vi "Settings_Config.vi"(11 "DataCluster in":T1={"Core"={"Current VI Reference"=refnum, "Close Panel on Exit?"=FALSE, "Exit"=FALSE, "Initialized?"=TRUE}, "Connections"={"cDAQ"={"Task"="", "Connected"=FALSE, "Active"=FALSE, "ID"="N/A"}, "Camera"={"Session"="", "Connected"=FALSE, "Active"=FALSE, "Placeholder"="remote image 00000211C32F1B68"}, "PSU"={"Port"="", "Connected"=FALSE, "Active"=FALSE}, "Arduino"={"Port"="", "Connected"=FALSE, "Active"=FALSE}}, "Data Acquisition"={"Setup"={"Label"="Sample_5", "Operator"="N/A", "Notes"="", "TempGrad"=-1.0, "TargetTemp"=-30.0, "Sample Volume"=1.0}, "Camera"={"Image"=refnum, "Save Image"=refnum, "Image Frequency"=20, "Rectangle"={"Left"=0, "Top"=0, "Right"=480, "Bottom"=620, "Rotation"=0.0}, "Calibration"={"Top Left"={"X"=62.0, "Y"=65.0}, "Top Right"={"X"=420.0, "Y"=58.0}, "Bottom Left"={"X"=67.0, "Y"=299.0}, "Bottom Right"={"X"=425.0, "Y"=292.0}, "Fixpoint"={"X"=469.0, "Y"=23.0}, "Scan Area"=5.0, "Fixpoint Area"=5.0, "Well Pixels"=array384x29[11136 elements], "Valid"=TRUE}, "FocusPos"=33419, "Display Mapping"=15, "Camera Mode"=10}, "Thermistor"={"Sample Size"=30, "Calibration"={"B0.100"=[3749.4, 3749.4, 3746.6, 3750.1, 3743.8, 3741.2, 3742.3, 3742.5], "R25"=[2.2631, 2.2631, 2.2535, 2.2652, 2.2631, 2.2501, 2.2549, 2.2676], "c"=[[-2.06472, 1.37415, -0.319461, 0.0344214, -0.0014593], [-2.06472, 1.37415, -0.319461, 0.0344214, -0.0014593], [-1.73592, 1.09563, -0.233459, 0.0229947, -0.0009224], [-2.12763, 1.40062, -0.319406, 0.0337046, -0.0014085], [-2.17313, 1.44996, -0.337063, 0.036201, -0.0015282], [-2.0427871, 1.4165762, -0.345474, 0.0385267, -0.0016538], [-2.1725266, 1.4989325, -0.3661616, 0.0412033, -0.0017892], [-2.2048521, 1.4601067, -0.3370514, 0.0360935, -0.0015259]], "State"=[FALSE, TRUE, TRUE, FALSE, TRUE, FALSE, FALSE, FALSE], "V_S"=12.004, "R_S"=10.0}, "Timing Mode"=14712}, "Partition"={"Data"=[["A", "35%", "", "", ""], ["B", "15%", "", "", ""], ["C", "5%", "", "", ""], ["D", "35%", "", "", ""], ["E", "Test sample", "", "", ""], ["F", "High Concentration", "", "", ""], ["G", "Low Concentration", "", "", ""], ["X", "Empty", "", "", ""]], "Cell Label"="A", "Cell Color"=29373, "Height"=10, "Width"=16, "Grid"=[]}, "Queue"={"Size"=10, "Queue"=refnum}, "Sample Rate"=120, "Active"=FALSE, "Ready"=TRUE, "Graph Mode"=0, "Gradient Buffer"=10}, "Control"={"Sample Rate"=1, "PID gains"={"proportional gain (Kc)"=6.485, "integral time (Ti, min)"=0.09, "derivative time (Td, min)"=0.03}}, "Manual Temp Control"={"TargetTemp"=1.0, "Mode"=0, "Active"=FALSE}} {"Manual Temp Control"."Mode" items=["Cool", "Heat"]; "Manual Temp Control"."TargetTemp" min=-40.0 max=40.0 step=0.5 format="%#_g °C"; "Control"."PID gains"."derivative time (Td, min)" format="%.3f"; "Control"."PID gains"."integral time (Ti, min)" format="%.3f"; "Control"."PID gains"."proportional gain (Kc)" format="%.3f"; "Control"."Sample Rate" min=1 max=20 step=1 format="%.0f Samples/sec"; "Data Acquisition"."Gradient Buffer" min=2 max=30 step=1; "Data Acquisition"."Graph Mode" items=["Thermistor Temperature", "Camera Temperature"]; "Data Acquisition"."Thermistor"."Timing Mode" items=["Automatic"=16097, "High Resolution"=10195, "High Speed"=14712, "Best 50 Hz Rejection"=14713, "Best 60 Hz Rejection"=14714, "Custom"=10137]; "Data Acquisition"."Thermistor"."Calibration"."R_S" min=0.1 max=1000.0 format="%#_g kOhm"; "Data Acquisition"."Thermistor"."Calibration"."V_S" min=5.0 max=48.0 format="%#_g V"; "Data Acquisition"."Thermistor"."Calibration"."R25" min=0.1 max=1000.0 format="%#_g kOhm"; "Data Acquisition"."Thermistor"."Calibration"."B0.100" min=100.0 max=10000.0 format="%#_g K"; "Data Acquisition"."Thermistor"."Sample Size" min=1 max=200; "Data Acquisition"."Sample Rate" min=20 max=240 format="%.0f samples/min"; "Data Acquisition"."Queue"."Size" min=1 max=200; "Data Acquisition"."Camera"."Camera Mode" items=["Temperature Linear", "Signal Linear"]; "Data Acquisition"."Camera"."Display Mapping" items=["Default"=10, "Most Significant Bits"=11, "Full Dynamic"=12, "Downshift"=13, "Given Range"=14, "90% Dynamic"=15, "Given Percent Range"=16]; "Data Acquisition"."Camera"."Calibration"."Fixpoint"."Y" format="%.2f"; "Data Acquisition"."Camera"."Calibration"."Fixpoint"."X" format="%.2f"; "Data Acquisition"."Camera"."Calibration"."Top Left"."Y" format="%.2f"; "Data Acquisition"."Camera"."Calibration"."Top Left"."X" format="%.2f"; "Data Acquisition"."Camera"."Calibration"."Top Right"."Y" format="%.2f"; "Data Acquisition"."Camera"."Calibration"."Top Right"."X" format="%.2f"; "Data Acquisition"."Camera"."Calibration"."Bottom Left"."Y" format="%.2f"; "Data Acquisition"."Camera"."Calibration"."Bottom Left"."X" format="%.2f"; "Data Acquisition"."Camera"."Calibration"."Bottom Right"."Y" format="%.2f"; "Data Acquisition"."Camera"."Calibration"."Bottom Right"."X" format="%.2f"; "Data Acquisition"."Camera"."Rectangle"."Rotation" min=-90.0 max=90.0 step=1.0 format="%.2f"; "Data Acquisition"."Camera"."Rectangle"."Left" scale=0.0..1024.0; "Data Acquisition"."Camera"."Rectangle"."Right" scale=0.0..1024.0; "Data Acquisition"."Camera"."Image Frequency" min=1 max=60 step=1; "Data Acquisition"."Setup"."Sample Volume" min=0.0 max=500.0 format="%#_g µL"; "Data Acquisition"."Setup"."TargetTemp" min=-40.0 max=40.0 step=0.5 format="%#_g °C"; "Data Acquisition"."Setup"."TempGrad" min=-100.0 max=100.0 step=0.1 format="%#_g °C/min"}) -> (0 "Canceled":bool, 3 "DataCluster out":T1={"Core"={"Current VI Reference"=refnum, "Close Panel on Exit?"=FALSE, "Exit"=FALSE, "Initialized?"=TRUE}, "Connections"={"cDAQ"={"Task"="", "Connected"=FALSE, "Active"=FALSE, "ID"="N/A"}, "Camera"={"Session"="", "Connected"=FALSE, "Active"=FALSE, "Placeholder"="remote image 00000211C32F1B68"}, "PSU"={"Port"="", "Connected"=FALSE, "Active"=FALSE}, "Arduino"={"Port"="", "Connected"=FALSE, "Active"=FALSE}}, "Data Acquisition"={"Setup"={"Label"="Sample_5", "Operator"="N/A", "Notes"="", "TempGrad"=-1.0, "TargetTemp"=-30.0, "Sample Volume"=1.0}, "Camera"={"Image"=refnum, "Save Image"=refnum, "Image Frequency"=20, "Rectangle"={"Left"=0, "Top"=0, "Right"=480, "Bottom"=620, "Rotation"=0.0}, "Calibration"={"Top Left"={"X"=62.0, "Y"=65.0}, "Top Right"={"X"=420.0, "Y"=58.0}, "Bottom Left"={"X"=67.0, "Y"=299.0}, "Bottom Right"={"X"=425.0, "Y"=292.0}, "Fixpoint"={"X"=469.0, "Y"=23.0}, "Scan Area"=5.0, "Fixpoint Area"=5.0, "Well Pixels"=array384x29[11136 elements], "Valid"=TRUE}, "FocusPos"=33419, "Display Mapping"=15, "Camera Mode"=10}, "Thermistor"={"Sample Size"=30, "Calibration"={"B0.100"=[3749.4, 3749.4, 3746.6, 3750.1, 3743.8, 3741.2, 3742.3, 3742.5], "R25"=[2.2631, 2.2631, 2.2535, 2.2652, 2.2631, 2.2501, 2.2549, 2.2676], "c"=[[-2.06472, 1.37415, -0.319461, 0.0344214, -0.0014593], [-2.06472, 1.37415, -0.319461, 0.0344214, -0.0014593], [-1.73592, 1.09563, -0.233459, 0.0229947, -0.0009224], [-2.12763, 1.40062, -0.319406, 0.0337046, -0.0014085], [-2.17313, 1.44996, -0.337063, 0.036201, -0.0015282], [-2.0427871, 1.4165762, -0.345474, 0.0385267, -0.0016538], [-2.1725266, 1.4989325, -0.3661616, 0.0412033, -0.0017892], [-2.2048521, 1.4601067, -0.3370514, 0.0360935, -0.0015259]], "State"=[FALSE, TRUE, TRUE, FALSE, TRUE, FALSE, FALSE, FALSE], "V_S"=12.004, "R_S"=10.0}, "Timing Mode"=14712}, "Partition"={"Data"=[["A", "35%", "", "", ""], ["B", "15%", "", "", ""], ["C", "5%", "", "", ""], ["D", "35%", "", "", ""], ["E", "Test sample", "", "", ""], ["F", "High Concentration", "", "", ""], ["G", "Low Concentration", "", "", ""], ["X", "Empty", "", "", ""]], "Cell Label"="A", "Cell Color"=29373, "Height"=10, "Width"=16, "Grid"=[]}, "Queue"={"Size"=10, "Queue"=refnum}, "Sample Rate"=120, "Active"=FALSE, "Ready"=TRUE, "Graph Mode"=0, "Gradient Buffer"=10}, "Control"={"Sample Rate"=1, "PID gains"={"proportional gain (Kc)"=6.485, "integral time (Ti, min)"=0.09, "derivative time (Td, min)"=0.03}}, "Manual Temp Control"={"TargetTemp"=1.0, "Mode"=0, "Active"=FALSE}} {"Manual Temp Control"."Mode" items=["Cool", "Heat"]; "Manual Temp Control"."TargetTemp" min=-40.0 max=40.0 step=0.5 format="%#_g °C"; "Control"."PID gains"."derivative time (Td, min)" format="%.3f"; "Control"."PID gains"."integral time (Ti, min)" format="%.3f"; "Control"."PID gains"."proportional gain (Kc)" format="%.3f"; "Control"."Sample Rate" min=1 max=20 step=1 format="%.0f Samples/sec"; "Data Acquisition"."Gradient Buffer" min=2 max=30 step=1; "Data Acquisition"."Graph Mode" items=["Thermistor Temperature", "Camera Temperature"]; "Data Acquisition"."Thermistor"."Timing Mode" items=["Automatic"=16097, "High Resolution"=10195, "High Speed"=14712, "Best 50 Hz Rejection"=14713, "Best 60 Hz Rejection"=14714, "Custom"=10137]; "Data Acquisition"."Thermistor"."Calibration"."R_S" min=0.1 max=1000.0 format="%#_g kOhm"; "Data Acquisition"."Thermistor"."Calibration"."V_S" min=5.0 max=48.0 format="%#_g V"; "Data Acquisition"."Thermistor"."Calibration"."R25" min=0.1 max=1000.0 format="%#_g kOhm"; "Data Acquisition"."Thermistor"."Calibration"."B0.100" min=100.0 max=10000.0 format="%#_g K"; "Data Acquisition"."Thermistor"."Sample Size" min=1 max=200; "Data Acquisition"."Sample Rate" min=20 max=240 format="%.0f samples/min"; "Data Acquisition"."Queue"."Size" min=1 max=200; "Data Acquisition"."Camera"."Camera Mode" items=["Temperature Linear", "Signal Linear"]; "Data Acquisition"."Camera"."Display Mapping" items=["Default"=10, "Most Significant Bits"=11, "Full Dynamic"=12, "Downshift"=13, "Given Range"=14, "90% Dynamic"=15, "Given Percent Range"=16]; "Data Acquisition"."Camera"."Calibration"."Fixpoint"."Y" format="%.2f"; "Data Acquisition"."Camera"."Calibration"."Fixpoint"."X" format="%.2f"; "Data Acquisition"."Camera"."Calibration"."Top Left"."Y" format="%.2f"; "Data Acquisition"."Camera"."Calibration"."Top Left"."X" format="%.2f"; "Data Acquisition"."Camera"."Calibration"."Top Right"."Y" format="%.2f"; "Data Acquisition"."Camera"."Calibration"."Top Right"."X" format="%.2f"; "Data Acquisition"."Camera"."Calibration"."Bottom Left"."Y" format="%.2f"; "Data Acquisition"."Camera"."Calibration"."Bottom Left"."X" format="%.2f"; "Data Acquisition"."Camera"."Calibration"."Bottom Right"."Y" format="%.2f"; "Data Acquisition"."Camera"."Calibration"."Bottom Right"."X" format="%.2f"; "Data Acquisition"."Camera"."Rectangle"."Rotation" min=-90.0 max=90.0 step=1.0 format="%.2f"; "Data Acquisition"."Camera"."Rectangle"."Left" scale=0.0..1024.0; "Data Acquisition"."Camera"."Rectangle"."Right" scale=0.0..1024.0; "Data Acquisition"."Camera"."Image Frequency" min=1 max=60 step=1; "Data Acquisition"."Setup"."Sample Volume" min=0.0 max=500.0 format="%#_g µL"; "Data Acquisition"."Setup"."TargetTemp" min=-40.0 max=40.0 step=0.5 format="%#_g °C"; "Data Acquisition"."Setup"."TempGrad" min=-100.0 max=100.0 step=0.1 format="%#_g °C/min"})   [LabVIEW 2024]
uses:
  DataCluster.ctl
  <vilib>/userDefined/High Color/IMAQdx.ctl
  <vilib>/vision/Image Controls.llb/IMAQ Image.ctl
panel:
  in  "Img_freq":u16(ring)=6 caption="Image Frequency" items=["60 img/min"=60, "30 img/min"=30, "20 img/min"=20, "15 img/min"=15, "12 img/min"=12, "10 img/min"=10, "6 img/min"=6]
  in  "Sample Volume":dbl=1.0 min=0.0 max=500.0 format="%#_g µL"
  in  "Target Temperature":dbl=-30.0 min=-30.0 max=40.0 step=0.5 format="%#_g °C"
  in  "OK":bool
  in  "Cancel":bool
  in  "Temperature Gradient":dbl=-1.0 min=-3.0 max=3.0 step=0.1 format="%#_g °C/min"
  in  "Notes":string
  in  "Operator":string="N/A"
  in  "Label":string="Sample_5"
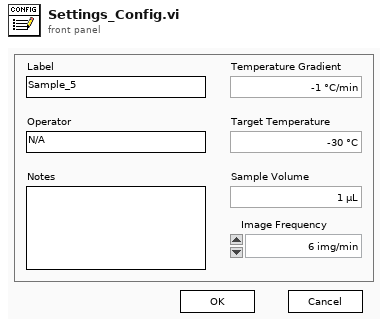
[diagram p1: front panel]
types:
  T1 = typedef "DataCluster.ctl" = cluster{"Core":cluster{"Current VI Reference":refnum<vi>, "Close Panel on Exit?":bool, "Exit":bool, "Initialized?":bool}, "Connections":cluster{"cDAQ":cluster{"Task":refnum<k21>, "Connected":bool, "Active":bool, "ID":string}, "Camera":cluster{"Session":T2, "Connected":bool, "Active":bool, "Placeholder":T3}, "PSU":cluster{"Port":refnum<visa-resource-name>, "Connected":bool, "Active":bool}, "Arduino":cluster{"Port":refnum<visa-resource-name>, "Connected":bool, "Active":bool}}, "Data Acquisition":cluster{"Setup":cluster{"Label":string, "Operator":string, "Notes":string, "TempGrad":dbl, "TargetTemp":dbl, "Sample Volume":dbl}, "Camera":cluster{"Image":T3, "Save Image":T3, "Image Frequency":i32, "Rectangle":T4, "Calibration":cluster{"Top Left":T5, "Top Right":T5, "Bottom Left":T5, "Bottom Right":T5, "Fixpoint":T5, "Scan Area":dbl, "Fixpoint Area":dbl, "Well Pixels":cluster{"X":i32, "Y":i32}[][], "Valid":bool}, "FocusPos":u32, "Display Mapping":u32, "Camera Mode":u32}, "Thermistor":cluster{"Sample Size":i32, "Calibration":cluster{"B0.100":dbl[], "R25":dbl[], "c":dbl[][], "State":bool[], "V_S":dbl, "R_S":dbl}, "Timing Mode":i32}, "Partition":cluster{"Data":string[][], "Cell Label":string, "Cell Color":u32, "Height":i32, "Width":i32, "Grid":string[][]}, "Queue":cluster{"Size":i32, "Queue":refnum<queue>}, "Sample Rate":i32, "Active":bool, "Ready":bool, "Graph Mode":u16, "Gradient Buffer":i32}, "Control":cluster{"Sample Rate":i32, "PID gains":cluster{"proportional gain (Kc)":dbl, "integral time (Ti, min)":dbl, "derivative time (Td, min)":dbl}}, "Manual Temp Control":cluster{"TargetTemp":dbl, "Mode":u16, "Active":bool}}
  T2 = typedef "IMAQdx.ctl" = refnum<k21>
  T3 = typedef "IMAQ Image.ctl" = refnum<image>
  T4 = typedef "IMAQ Rectangle" = cluster{"Left":i32, "Top":i32, "Right":i32, "Bottom":i32, "Rotation":dbl}
  T5 = typedef "IMAQ Point" = cluster{"X":sgl, "Y":sgl}
  T6 = enum8{"Enabled", "Disabled", "Disabled and Grayed Out"}
  T7 = cluster{"Label":string, "Operator":string, "Notes":string, "TempGrad":dbl, "TargetTemp":dbl, "Sample Volume":dbl}
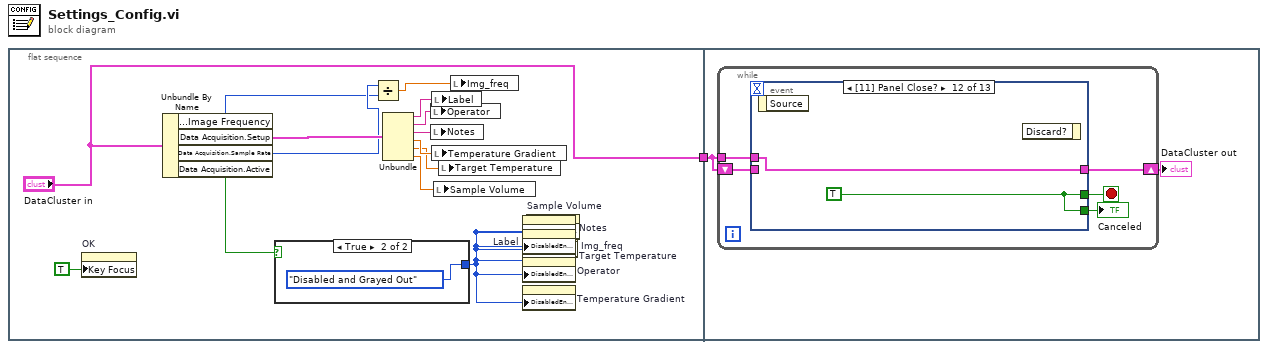
[diagram p0: block diagram]
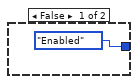
[diagram p2: hidden frame]
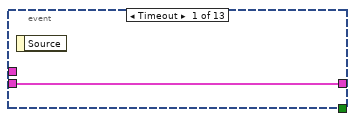
[diagram p3: hidden frame]
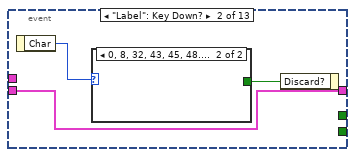
[diagram p4: hidden frame]
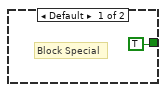
[diagram p5: hidden frame]
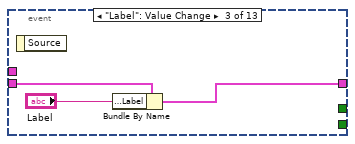
[diagram p6: hidden frame]
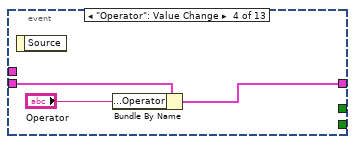
[diagram p7: hidden frame]
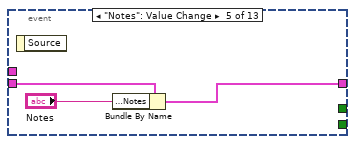
[diagram p8: hidden frame]
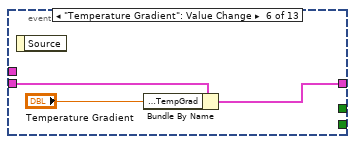
[diagram p9: hidden frame]
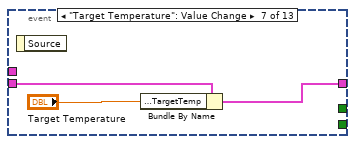
[diagram p10: hidden frame]
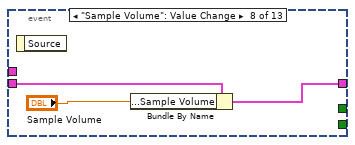
[diagram p11: hidden frame]
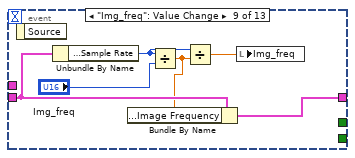
[diagram p12: hidden frame]
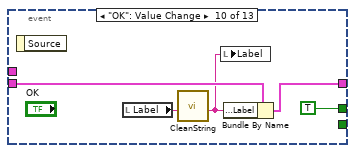
[diagram p13: hidden frame]
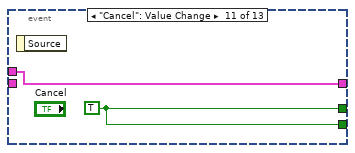
[diagram p14: hidden frame]
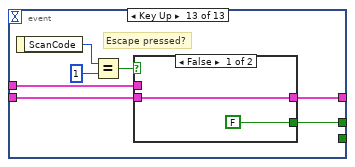
[diagram p15: hidden frame]
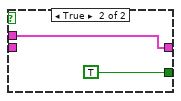
[diagram p16: hidden frame]
diagram:
  n1 = flat-sequence {
    tunnel: ["DataCluster in"] -> w1
    tunnel: w1 -> [w19]
    frame #0 {
      n2 = property on="OK" class="Bool"("Key Focus"=TRUE) -> ()  [unwired: 2 in, 2 out]
      n3 = Unbundle By Name("DataCluster in") -> ("Data Acquisition.Camera.Image Frequency"=w4:i32, "Data Acquisition.Setup"=w15:T7, "Data Acquisition.Sample Rate"=w5:i32, "Data Acquisition.Active"=w8:bool)
      n4 = case shown="True" w8 {
        tunnel: [T6."Enabled" ("Disabled") T6."Disabled and Grayed Out" ("Disabled")] -> w2
        frame False {
        }
        frame True {
        }
      }
      n5 = Divide(x=w5, y=w4) -> (x/y=w3:dbl)
      n6 = Unbundle(w15) -> ("Label"=w14:string, "Operator"=w10:string, "Notes"=w9:string, "TempGrad"=w13:dbl, "TargetTemp"=w6:dbl, "Sample Volume"=w7:dbl)
      n7 = local write "Operator"(w10) -> ()
      n8 = local write "Notes"(w9) -> ()
      n9 = local write "Label"(w14) -> ()
      n10 = local write "Temperature Gradient"(w13) -> ()
      n11 = local write "Sample Volume"(w7) -> ()
      n12 = local write "Target Temperature"(w6) -> ()
      n13 = local write "Img_freq"(w3) -> ()
      n14 = property on="Notes" class="Str"("DisabledEnum"=w2) -> ()  [unwired: 2 in, 2 out]
      n15 = property on="Label" class="Str"("DisabledEnum"=w2) -> ()  [unwired: 2 in, 2 out]
      n16 = property on="Target Temperature" class="DigNum (strict)"("DisabledEnum"=w2) -> ()  [unwired: 2 in, 2 out]
      n17 = property on="Operator" class="Str"("DisabledEnum"=w2) -> ()  [unwired: 2 in, 2 out]
      n18 = property on="Temperature Gradient" class="DigNum (strict)"("DisabledEnum"=w2) -> ()  [unwired: 2 in, 2 out]
      n19 = property on="Img_freq" class="Ring (strict)"("DisabledEnum"=w2) -> ()  [unwired: 2 in, 2 out]
      n20 = property on="Sample Volume" class="DigNum (strict)"("DisabledEnum"=w2) -> ()  [unwired: 2 in, 2 out]
    }
    frame #1 {
      n21 = while {
        shift-right: [w24] -> w18
        shift-left: w19 -> [w23]
        tunnel: w19 -> [w22]
        stop <- w21 stop-if-true
        n22 = event shown="[11] Panel Close?" {
          selector: _ -> [_ _ _ _ _ _ _ _ _ _ _ _ _]
          dyn-events: _ -> [_ _ _ _ _ _ _ _ _ _ _ _ _]
          timeout: _ -> [_ _ _ _ _ _ _ _ _ _ _ _ _]
          tunnel: w23 -> [w25 w26 w32 w35 w38 w41 w44 w47 w52 w56 _ _ w63]
          tunnel: [w25 w26 w31 w34 w37 w40 w43 w46 w53 w55 w60 w62 w65] -> w24
          tunnel: w22 -> [_ _ _ _ _ _ _ _ _ _ w60 w62 w64]
          tunnel: [_ _ _ _ _ _ _ _ _ TRUE w59 w61 w69] -> w21
          tunnel: [_ _ _ _ _ _ _ _ _ _ w59 w61 _] -> w20
          event Timeout {
            n23 = event-data() -> ()  [unwired: 1 in, 1 out]
          }
          event "Label": Key Down? {
            n24 = event-data() -> ("Char"=w28:i16)  [unwired: 1 in]
            n25 = case shown="0, 8, 32, 43, 45, 48..57, 65..90, 95, 97..122" w28 {
              tunnel: [TRUE _] -> w27
              frame Default {
                # "Block Special"
              }
              frame 0, 8, 32, 43, 45, 48..57, 65..90, 95, 97..122 {
              }
            }
            n26 = event-data("Discard?"=w27) -> ()  [unwired: 1 in, 1 out]
          }
          event "Label": Value Change {
            n27 = event-data() -> ()  [unwired: 1 in, 1 out]
            n28 = Bundle By Name(cluster=w32, "Data Acquisition.Setup.Label"="Label") -> (w31:T1)
          }
          event "Operator": Value Change {
            n29 = event-data() -> ()  [unwired: 1 in, 1 out]
            n30 = Bundle By Name(cluster=w35, "Data Acquisition.Setup.Operator"="Operator") -> (w34:T1)
          }
          event "Notes": Value Change {
            n31 = event-data() -> ()  [unwired: 1 in, 1 out]
            n32 = Bundle By Name(cluster=w38, "Data Acquisition.Setup.Notes"="Notes") -> (w37:T1)
          }
          event "Temperature Gradient": Value Change {
            n33 = event-data() -> ()  [unwired: 1 in, 1 out]
            n34 = Bundle By Name(cluster=w41, "Data Acquisition.Setup.TempGrad"="Temperature Gradient") -> (w40:T1)
          }
          event "Target Temperature": Value Change {
            n35 = event-data() -> ()  [unwired: 1 in, 1 out]
            n36 = Bundle By Name(cluster=w44, "Data Acquisition.Setup.TargetTemp"="Target Temperature") -> (w43:T1)
          }
          event "Sample Volume": Value Change {
            n37 = event-data() -> ()  [unwired: 1 in, 1 out]
            n38 = Bundle By Name(cluster=w47, "Data Acquisition.Setup.Sample Volume"="Sample Volume") -> (w46:T1)
          }
          event "Img_freq": Value Change {
            n39 = event-data() -> ()  [unwired: 1 in, 1 out]
            n40 = Unbundle By Name(w52) -> ("Data Acquisition.Sample Rate"=w50:i32)
            n41 = Divide(x=w50, y="Img_freq") -> (x/y=w51:dbl)
            n42 = Bundle By Name(cluster=w52, "Data Acquisition.Camera.Image Frequency"=w51) -> (w53:T1)
            n43 = Divide(x=w50, y=w51) -> (x/y=w49:dbl)
            n44 = local write "Img_freq"(w49) -> ()
          }
          event "OK": Value Change {
            n45 = event-data() -> ()  [unwired: 1 in, 1 out]
            n46 = local read "Label"() -> (w57:string)
            n47 = call "CleanString.vi"("Input"=w57) -> ("Cleaned"=w54:string)  [unwired: 8 in]
            n48 = local write "Label"(w54) -> ()
            n49 = Bundle By Name(cluster=w56, "Data Acquisition.Setup.Label"=w54) -> (w55:T1)
          }
          event "Cancel": Value Change {
            w59 = TRUE
            n50 = event-data() -> ()  [unwired: 1 in, 1 out]
          }
          event Panel Close? {
            w61 = TRUE
            n51 = event-data() -> ()  [unwired: 1 in, 1 out]
            n52 = event-data() -> ()  [unwired: 2 in, 1 out]
          }
          event Key Up {
            # "Escape pressed?"
            n53 = event-data() -> ("ScanCode"=w68:i16)  [unwired: 1 in]
            n54 = Equal?(x=w68, y=i16 1) -> (x = y?=w66:bool)
            n55 = case shown="False" w66 {
              tunnel: [FALSE TRUE] -> w69
              tunnel: [w71 w72] -> w65
              tunnel: w64 -> [_ w72]
              tunnel: w63 -> [w71 _]
              frame False {
              }
              frame True {
              }
            }
          }
        }
        "Canceled" <- w20
      }
      "DataCluster out" <- w18
    }
  }
